vi "Create Reservation Annotations.vi"(8 "error in":errorcluster) -> (0 "error out":errorcluster, 3 "annotations array":T1[](array[typedef]))   [LabVIEW 2021, in "NI Session Management V1 Client.lvlib" / "Session Reservation.lvclass"]
uses:
  Session Reservation.lvclass
  gRPC/Generated APIs/ni/measurementlink/sessionmanagement/v1/RPC Messages/ni_measurementlink_sessionmanagement_v1_SessionInformation_AnnotationsEntry.ctl
  96ebd3b6-2171-43d4-b6b2-fee63be2a44d.vi
  Get Client Machine Details.vi
  Session Reservation.lvclass/Session Reservation.ctl
  gRPC/Generated APIs/ni/measurementlink/sessionmanagement/v1/ni.measurementlink.sessionmanagement.v1.api.lvlib
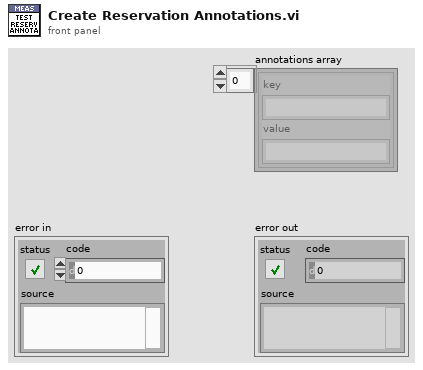
[diagram p1: front panel]
types:
  T1 = typedef "ni.measurementlink.sessionmanagement.v1.api.lvlib/ni_measurementlink_sessionmanagement_v1_SessionInformation_AnnotationsEntry.ctl" = cluster{"key":string, "value":string}
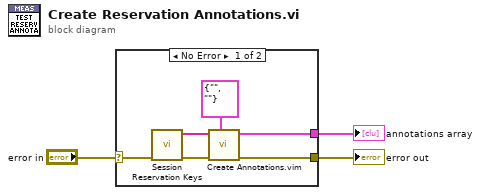
[diagram p0: block diagram]
diagram:
  n1 = case shown="No Error" "error in" {
    selector: "error in" -> [w7 w9]
    tunnel: [w4 _] -> w3
    tunnel: [w6 w9] -> w1
    frame No Error {
      n2 = call "Session Reservation Keys.vi"() -> ("session reservation keys"=w5:string[])  [unwired: 11 in]
      n3 = call "Create Annotations.vim"("annotation typedef"=T1 {"key"="", "value"=""} ("ni_measurementlink_sessionmanagement_v1_SessionInformation_AnnotationsEntry"), "error in"=w7, "annotation keys"=w5) -> ("error out"=w6:errorcluster, "annotations array"=w4:T1[])  [unwired: 7 in]
    }
    frame Error {
    }
  }
  "annotations array" <- w3
  "error out" <- w1
